vi "VI Pop Up.vi"(7 "Aufrufer gesperrt?":bool, 8 "Fehler (Eingang, kein Fehler)":errorcluster, 9 "Warten bis beendet":bool, 11 "VI Referenz":refnum<vi>) -> (0 "Fehler (Ausgang)":errorcluster)   [LabVIEW 2020]
panel:
  out "Referenz (Ausgang)":refnum<vi>
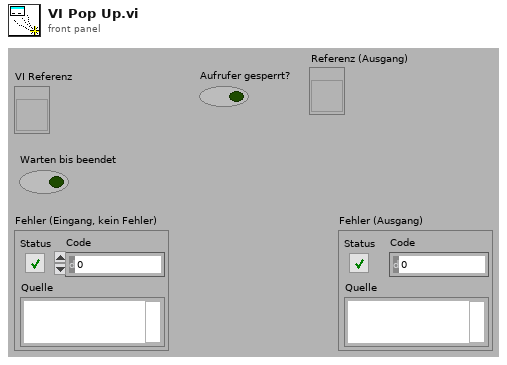
[diagram p1: front panel]
types:
  T1 = enum32{"Invalid", "Default", "Floating", "Floating/Auto-Hide", "Modal"}
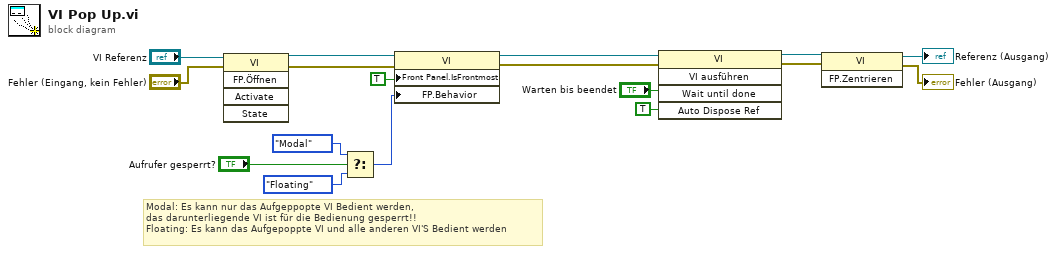
[diagram p0: block diagram]
diagram:
  # "Modal: Es kann nur das Aufgeppopte VI Bedient werden, \ndas darunterliegende VI ist für die Bedienung gesperrt!!\nFloating: Es kann das Aufgepoppte VI und alle anderen VI'S Bedient werden"
  n1 = invoke class="VI" method="FP.Öffnen"(reference="VI Referenz", error in="Fehler (Eingang, kein Fehler)") -> (reference out=w8:refnum<vi>, error out=w11:errorcluster)  [unwired: 3 in, 3 out]
  n2 = Select(t=T1."Modal" ("Frontpanel-Fenster:Verhaltensweise"), s="Aufrufer gesperrt?", f=T1."Floating" ("Frontpanel-Fenster:Verhaltensweise")) -> (s? t:f=w12:T1)
  n3 = property class="VI"(reference=w8, error in=w11, "Front Panel.IsFrontmost"=TRUE ("Frontpanel-Fenster:Ist im Vordergrund"), "FP.Behavior"=w12) -> (reference out=w7:refnum<vi>, error out=w10:errorcluster)
  n4 = invoke class="VI" method="VI ausführen"(reference=w7, error in=w10, "Wait until done"="Warten bis beendet", "Auto Dispose Ref"=TRUE ("Referenz automatisch schließen")) -> (reference out=w6:refnum<vi>, error out=w9:errorcluster)  [unwired: 1 in, 3 out]
  n5 = invoke class="VI" method="FP.Zentrieren"(reference=w6, error in=w9) -> (reference out=→"Referenz (Ausgang)":refnum<vi>, error out=→"Fehler (Ausgang)":errorcluster)  [unwired: 1 in, 1 out]
